vi "target menu name.vi"(8 "error in":errorcluster, 11 "PLTarget PC in":refnum<class "PLTarget PC.lvclass">) -> (0 "error out":errorcluster, 2 "menu name":string, 3 "PLTarget PC out":refnum<class "PLTarget PC.lvclass">)   [LabVIEW 2013, in "PLTarget PC.lvclass"]
uses:
  PLTarget PC.lvclass
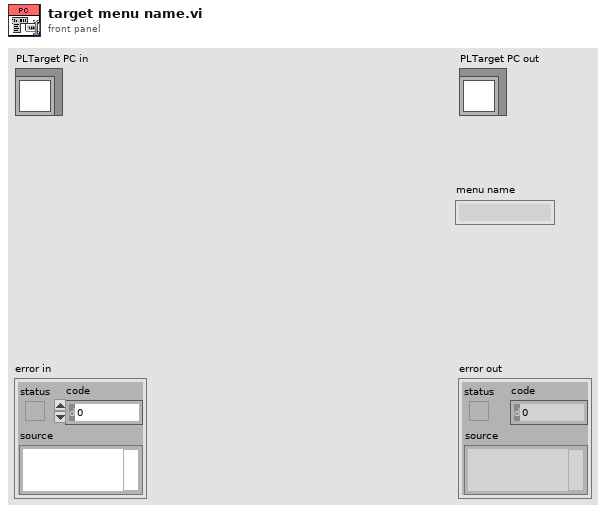
[diagram p1: front panel]
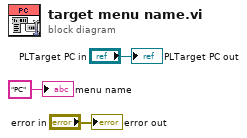
[diagram p0: block diagram]
diagram:
  "error out" <- "error in"
  "PLTarget PC out" <- "PLTarget PC in"
  "menu name" <- "PC" ("menu name")
